vi "Send Message.vi"(8 "error in (no error)":errorcluster, 9 "Value":dbl, 10 "Message to Send":T1, 11 "Oven in":refnum<class "Oven.lvclass">) -> (0 "error out":errorcluster, 3 "Oven out":refnum<class "Oven.lvclass">)   [LabVIEW 2018, in "Oven.lvlib" / "Oven.lvclass"]
uses:
  Oven.lvclass
  Custom Controls/Message Type.ctl
  Oven.lvlib
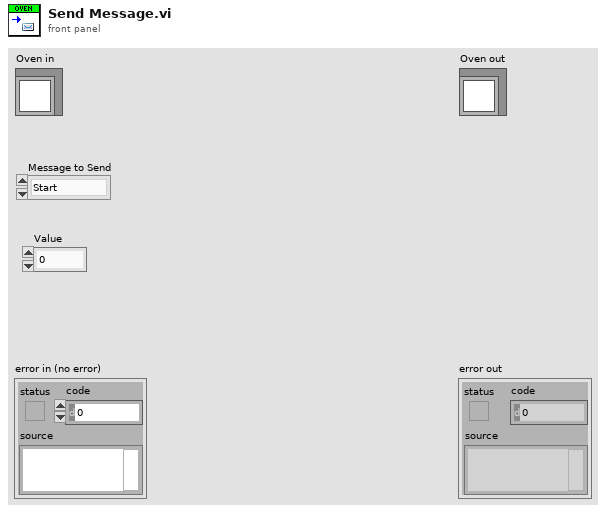
[diagram p1: front panel]
types:
  T1 = typedef "Oven.lvlib/Message Type.ctl" = enum16{"Start", "Stop", "Set Temperature", "Get Temperature"}
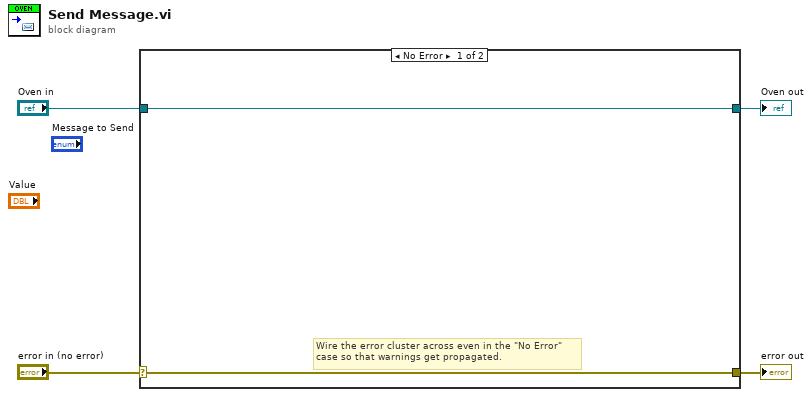
[diagram p0: block diagram]
diagram:
  n1 = case shown="No Error" "error in (no error)" {
    selector: "error in (no error)" -> [w5 w8]
    tunnel: [w5 w8] -> w3
    tunnel: [w6 w7] -> w1
    tunnel: "Oven in" -> [w6 w7]
    frame No Error {
      # "Wire the error cluster across even in the \"No Error\"\ncase so that warnings get propagated."
    }
    frame Error {
    }
  }
  "error out" <- w3
  "Oven out" <- w1
